vi "HNE Page Manager (Set).vi"(3 "error in (no error)":errorcluster, 4 "Next Page":string) -> (0 "error out":errorcluster)   [LabVIEW 2013]
doc: "This VI writes the name of the next page to be displayed to the page manager"
uses:
  _SubVIs/TypeDefs/Page Operation.ctl
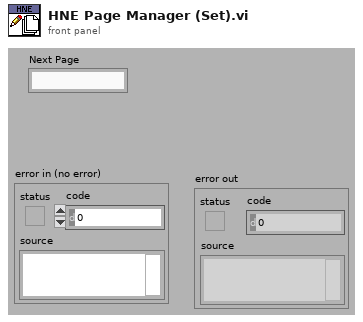
[diagram p1: front panel]
types:
  T1 = typedef "Page Operation.ctl" = enum16{"Init", "Set Next", "Get Next", "Back"}
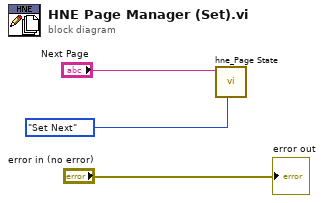
[diagram p0: block diagram]
diagram:
  n1 = call "hne_Page State.vi"("Page Operation"=Page_Operation."Set Next", "Next Page"="Next Page") -> ()  [unwired: 2 in, 8 out]
  "error out" <- "error in (no error)"
